vi "ReadPersistentConfiguration.vi"(8 "Error In":errorcluster, 10 "DataIn":variant, 11 "OpenCVCam in":refnum<class "OpenCVCam.lvclass">) -> (0 "Error Out":errorcluster, 2 "DataOut":variant, 3 "OpenCVCam out":refnum<class "OpenCVCam.lvclass">)   [LabVIEW 2021, in "OpenCVCam.lvclass"]
uses:
  OpenCVCam.lvclass
  OpenCVCam.lvclass/OpenCVCam.ctl
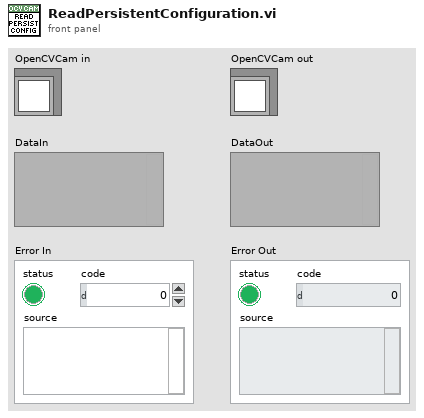
[diagram p1: front panel]
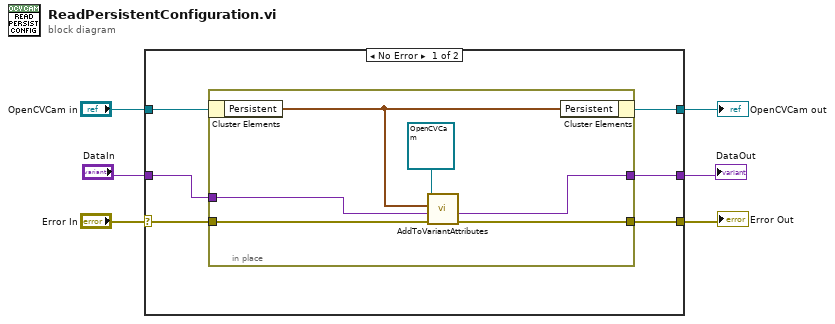
[diagram p0: block diagram]
diagram:
  n1 = case shown="No Error" "Error In" {
    selector: "Error In" -> [w10 w21]
    tunnel: [w9 w21] -> w5
    tunnel: [w7 w20] -> w3
    tunnel: "OpenCVCam in" -> [w12 w20]
    tunnel: "DataIn" -> [w11 w19]
    tunnel: [w8 w19] -> w1
    frame No Error {
      n2 = in-place {
        in-place-border: [w17] -> w9
        in-place-border: w11 -> [w16]
        in-place-border: [w15] -> w8
        in-place-border: w10 -> [w18]
        n3 = in-place-cluster #1(w12) -> ("Persistent"=w13:cluster{"Dummy":dbl})
        n4 = call "AddToVariantAttributes.vi"("error in (no error)"=w18, "DataIn in"=w16, "PersistentData"=w13, "Object"=refnum<class "OpenCVCam.lvclass"> refnum ("ApplicationGUI2")) -> ("error out"=w17:errorcluster, "DataIn out"=w15:variant)  [unwired: 6 in]
        n5 = in-place-cluster #1("Persistent"=w13) -> (w7:refnum<class "OpenCVCam.lvclass">)
      }
    }
    frame Error {
    }
  }
  "Error Out" <- w5
  "OpenCVCam out" <- w3
  "DataOut" <- w1
